vi "Configure Gate Time.vi"(0 "VISA resource name":refnum<visa-resource-name>, 1 "Enable Gate (T: Enable)":bool=TRUE, 2 "Gate Length (1E-6 s)":dbl=1e-06, 3 "Level (0: High)":u16(ring) items=["High", "Low"], 5 "Gate Control (0: Edge)":u16(ring) items=["Edge", "Level"], 7 "Slope (0: Negative)":u16(ring) items=["Negative", "Positive"], 9 "Gate Delay (1E-6 s)":dbl=1e-06, 11 "error in (no error)":errorcluster) -> (4 "VISA resource name out":refnum<visa-resource-name>, 15 "error out":errorcluster)   [LabVIEW 2014, in "Agilent ESA PSA Series.lvlib"]
doc: "Configures Time Gate.\n\n<B>Note:</B>\n\nThis function is available only when option 1D6 is installed."
uses:
  Agilent ESA PSA Series.lvlib
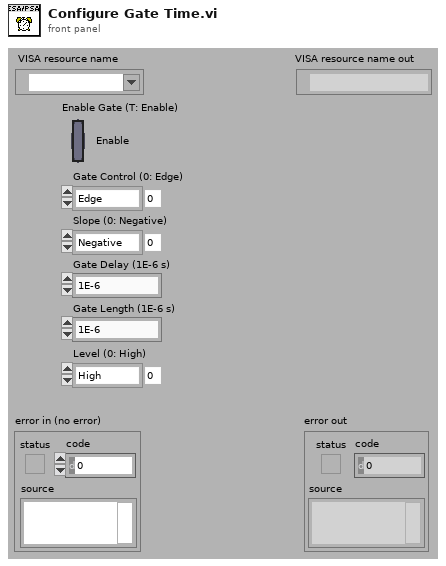
[diagram p1: front panel]
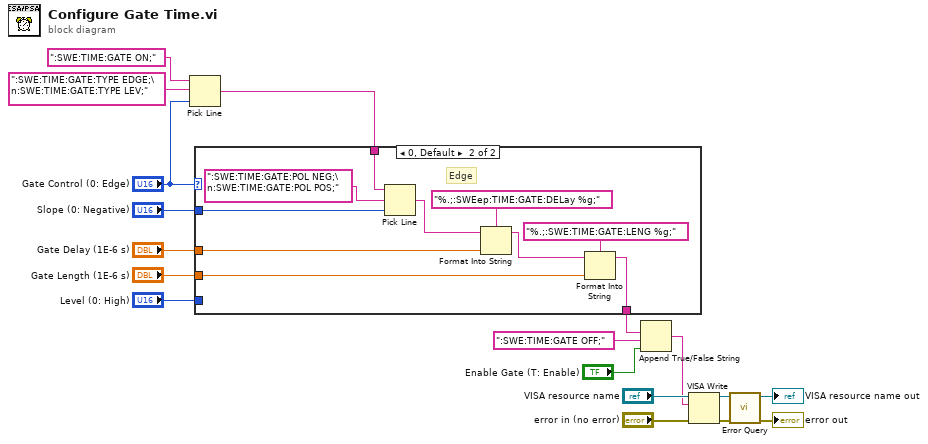
[diagram p0: block diagram]
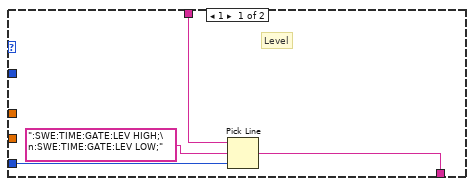
[diagram p2: hidden frame]
diagram:
  n1 = Pick Line(string ("")=":SWE:TIME:GATE ON;", multi-line string=":SWE:TIME:GATE:TYPE EDGE;\n:SWE:TIME:GATE:TYPE LEV;", line index="Gate Control (0: Edge)") -> (output string=w3:string)
  n2 = case shown="0, Default" "Gate Control (0: Edge)" {
    tunnel: "Slope (0: Negative)" -> [_ w31]
    tunnel: "Gate Delay (1E-6 s)" -> [_ w28]
    tunnel: "Gate Length (1E-6 s)" -> [_ w25]
    tunnel: w3 -> [w20 w24]
    tunnel: "Level (0: High)" -> [w21 _]
    tunnel: [w19 w23] -> w1
    frame 1 {
      # "Level"
      n3 = Pick Line(string ("")=w20, multi-line string=":SWE:TIME:GATE:LEV HIGH;\n:SWE:TIME:GATE:LEV LOW;", line index=w21) -> (output string=w19:string)
    }
    frame 0, Default {
      # "Edge"
      n4 = Pick Line(string ("")=w24, multi-line string=":SWE:TIME:GATE:POL NEG;\n:SWE:TIME:GATE:POL POS;", line index=w31) -> (output string=w30:string)
      n5 = Format Into String(format string="%.;:SWEep:TIME:GATE:DELay %g;", initial string=w30, w28) -> (resulting string=w26:string)  [unwired: 1 in, 1 out]
      n6 = Format Into String(format string="%.;:SWE:TIME:GATE:LENG %g;", initial string=w26, w25) -> (resulting string=w23:string)  [unwired: 1 in, 1 out]
    }
  }
  n7 = Append True/False String(1:"Enable Gate (T: Enable)", 2:":SWE:TIME:GATE OFF;" ("false string"), 3:w1) -> (0:w12:string)  [unwired: 1 in]
  n8 = VISA Write(VISA resource name="VISA resource name", write buffer=w12, error in (no error)="error in (no error)") -> (VISA resource name out=w16:refnum<visa-resource-name>, error out=w14:errorcluster)  [unwired: 1 out]
  n9 = call "Error Query.vi"("error in (no error)"=w14, "VISA resource name"=w16) -> ("error out"=→"error out":errorcluster, "VISA resource name out"=→"VISA resource name out":refnum<visa-resource-name>)  [unwired: 6 in, 2 out]
